vi "Add_Positions_to_stats.vi"(8 "Data row":string[](array[string]), 9 "No of stats columns":i32[](array[numeric]), 10 "Position":T1(array[cluster])=[{"Name"="LDA", "X"=999.9865969709155, "Y"=0.004861094232311693, "Z"=40.00084175084175}, {"Name"="CW", "X"=999.9865969709155, "Y"=0.004861094232311693, "Z"=40.00084175084175}, {"Name"="Gen", "X"=-2000.0, "Y"=200.0, "Z"=980.0}, {"Name"="T", "X"=999.9865969709155, "Y"=0.004861094232311693, "Z"=40.00084175084175}] {"Z" format="%.1f"; "Y" format="%.1f"; "X" format="%.1f"}) -> (0 "Data row with positions":string[](array[string]), 3 "row splitting":string[][](array[string]))   [LabVIEW 2010]
uses:
  Globals/Meas_global.vi
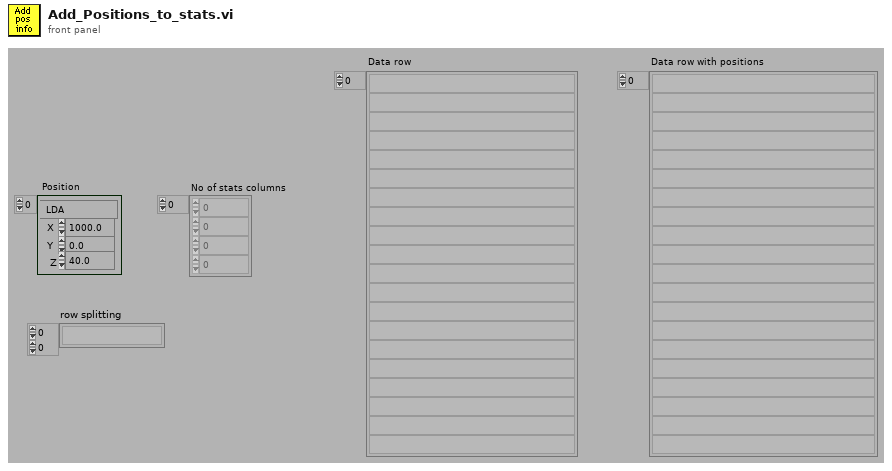
[diagram p1: front panel]
types:
  T1 = cluster{"Name":string, "X":dbl, "Y":dbl, "Z":dbl}[]
  T2 = cluster{"Name":string, "X":dbl, "Y":dbl, "Z":dbl}
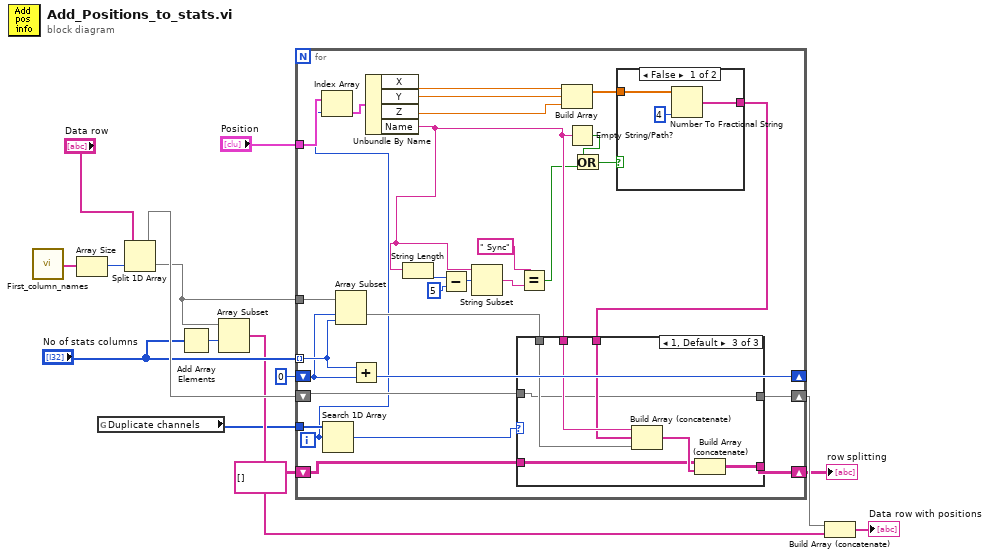
[diagram p0: block diagram]
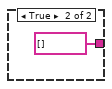
[diagram p2: hidden frame]
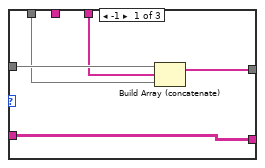
[diagram p3: hidden frame]
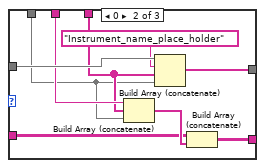
[diagram p4: hidden frame]
diagram:
  n1 = call "First_column_names.vi"() -> ("Array"=w4:string[])
  n2 = Array Size(array=w4) -> (size(s)=w12:i32)
  n3 = global read "Meas_global.vi" "Duplicate channels"() -> (w1:i32[])
  n4 = Split 1D Array(array="Data row", index=w12) -> (first subarray=w11:string[], second subarray=w6:string[])
  n5 = Add Array Elements(numeric array="No of stats columns") -> (sum=w7:i32)
  n6 = Array Subset(array=w6, index=w7) -> (w5:string[])  [unwired: 1 in]
  n7 = for {
    shift-right: [w41] -> w8
    shift-left: w11 -> [w42]
    tunnel: "Position" -> [w27]
    tunnel: "No of stats columns" -> [w40] mode=indexing
    tunnel: w6 -> [w43]
    shift-right: [w39] -> _
    shift-left: 0 -> [w38]
    tunnel: w1 -> [w31]
    shift-right: [w29] -> w2
    shift-left: string[][] [] -> [w28]
    i -> [w26]
    n8 = Index Array(array=w27, index=w26) -> (element=w25:T2)
    n9 = Search 1D Array(1D array=w31, element=w26) -> (index of element=w30:i32)  [unwired: 1 out]
    n10 = Array Subset(array=w43, index=w38, length=w40) -> (w33:string[])
    n11 = Add(x=w40, y=w38) -> (x+y=w39:i32)
    n12 = Unbundle By Name(w25) -> ("X"=w35:dbl, "Y"=w36:dbl, "Z"=w37:dbl, "Name"=w17:string)
    n13 = String Length(string=w17) -> (length=w22:i32)
    n14 = Subtract(x=w22, y=5) -> (x-y=w21:i32)
    n15 = String Subset(string=w17, offset (0)=w21) -> (substring=w19:string)  [unwired: 1 out]
    n16 = Equal?(x=" Sync" ("substring"), y=w19) -> (x = y?=w16:bool)
    n17 = Build Array(w35, w36, w37) -> (w34:dbl[])
    n18 = Empty String/Path?(string/path=w17) -> (empty?=w24:bool)
    n19 = Or(x=w24, y=w16) -> (x .or. y?=w23:bool)
    n20 = case shown="False" w23 {
      tunnel: w34 -> [w45 _]
      tunnel: [w44 string[] []] -> w32
      frame False {
        n21 = Number To Fractional String(number=w45, precision (6)=i16 4) -> (F-format string=w44:string[])  [unwired: 2 out]
      }
      frame True {
      }
    }
    n22 = case shown="1, Default" w30 {
      tunnel: w42 -> [w52 w60 w62]
      tunnel: [w51 w61 w62] -> w41
      tunnel: w33 -> [w50 w56 w66]
      tunnel: w32 -> [w49 w57 w67]
      tunnel: w17 -> [_ w58 w68]
      tunnel: [w48 w54 w64] -> w29
      tunnel: w28 -> [w48 w53 w63]
      frame -1 {
        n23 = Build Array (concatenate)(w52, w49, w50) -> (w51:string[])
      }
      frame 0 {
        n24 = Build Array (concatenate)(w58, w57, w56) -> (w55:string[])
        n25 = Build Array (concatenate)(w60, "Instrument_name_place_holder", w57, w56) -> (w61:string[])
        n26 = Build Array (concatenate)(w53, w55) -> (w54:string[][])
      }
      frame 1, Default {
        n27 = Build Array (concatenate)(w68, w67, w66) -> (w65:string[])
        n28 = Build Array (concatenate)(w63, w65) -> (w64:string[][])
      }
    }
  }
  "row splitting" <- w2
  n29 = Build Array (concatenate)(w8, w5) -> (→"Data row with positions":string[])
